vi "FP-BoundSV.vi"() -> ()   [LabVIEW 2020, in "BNT_DAQmx.lvlib"]
uses:
  BNT_DAQmx.lvlib
panel:
  out "DI":bool[](array[boolean])
  out "AI":dbl[](array[numeric])
  out "DO":bool[](array[boolean])
  out "AO":dbl[](array[numeric])
  in  "Set-DO":bool[](array[boolean])
  in  "Set-AO":dbl[](array[numeric])
  in  "Stop Button":bool
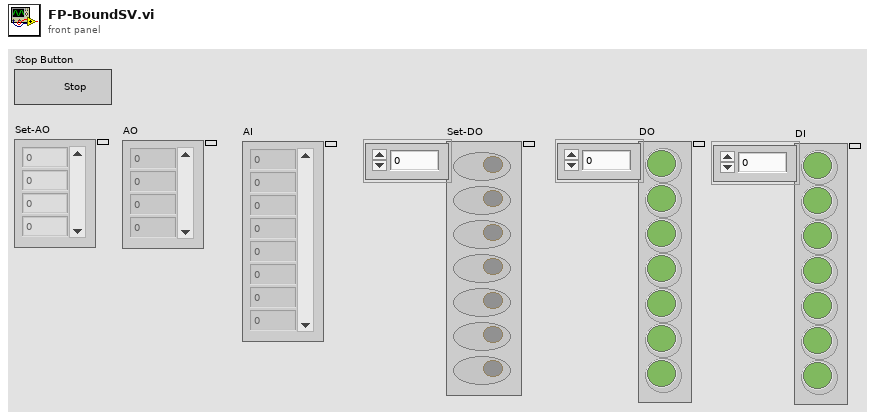
[diagram p1: front panel]
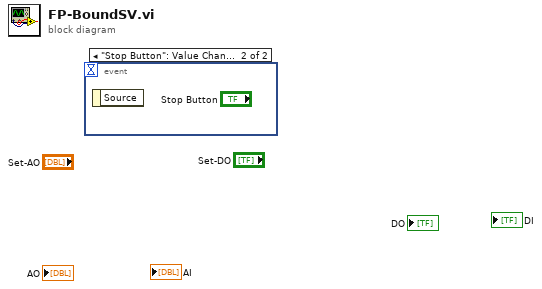
[diagram p0: block diagram]
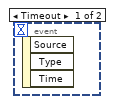
[diagram p2: hidden frame]
diagram:
  n1 = event shown="[1] \"Stop Button\": Value Change" {
    selector: _ -> [_ _]
    dyn-events: _ -> [_ _]
    timeout: _ -> [_ _]
    event Timeout {
      n2 = event-data() -> ()  [unwired: 1 in, 3 out]
    }
    event "Stop Button": Value Change {
      n3 = event-data() -> ()  [unwired: 1 in, 1 out]
    }
  }
